vi "LogMessage.vi"(0 "GenericCanAdapterClass in":refnum<class "GenericCanAdapterClass.lvclass">, 1 "LogSuspend":bool, 3 "Name":string, 5 "Arbitration Id":u32 format="%08x", 7 "DataLength":u8, 9 "Data":u8[](array[numeric]) format="%02x", 11 "error in":errorcluster) -> (4 "GenericCanAdapterClass out":refnum<class "GenericCanAdapterClass.lvclass">, 15 "error out":errorcluster)   [LabVIEW 2011, in "GenericCanAdapterClass.lvclass"]
uses:
  GenericCanAdapterClass.lvclass
  GenericCanAdapterClass.lvclass/GenericCanAdapterClass.ctl
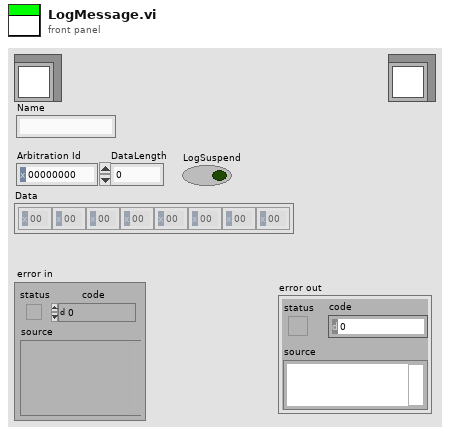
[diagram p1: front panel]
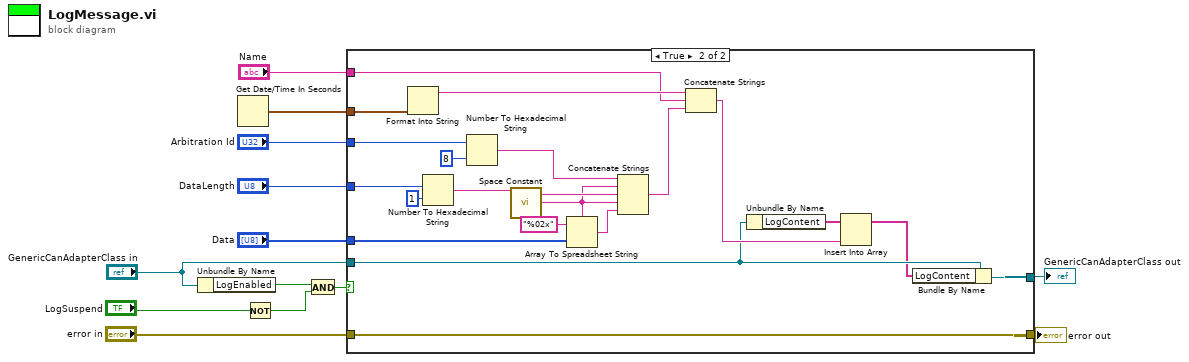
[diagram p0: block diagram]
diagram:
  n1 = Unbundle By Name("GenericCanAdapterClass in") -> ("LogEnabled"=w8:bool)
  n2 = Get Date/Time In Seconds() -> (seconds since 1Jan1904=w13:timestamp)
  n3 = Not(x="LogSuspend") -> (.not. x?=w10:bool)
  n4 = And(x=w8, y=w10) -> (x .and. y?=w11:bool)
  n5 = case shown="True" w11 {
    tunnel: "error in" -> [w15 w22]
    tunnel: [w15 w22] -> w5
    tunnel: [w14 w19] -> w2
    tunnel: "GenericCanAdapterClass in" -> [w14 w18]
    tunnel: "Data" -> [_ w29]
    tunnel: "DataLength" -> [_ w28]
    tunnel: "Arbitration Id" -> [_ w26]
    tunnel: w13 -> [_ w24]
    tunnel: "Name" -> [_ w16]
    frame False {
    }
    frame True {
      n6 = Format Into String(w24) -> (resulting string=w23:string)  [unwired: 3 in, 1 out]
      n7 = Number To Hexadecimal String(1:i16 1 ("width (-)"), 2:w28) -> (0:w35:string)
      n8 = Number To Hexadecimal String(1:i16 8 ("width (-)"), 2:w26) -> (0:w25:string)
      n9 = call <vilib>:"Space Constant.vi"() -> ("String"=w33:string)
      n10 = Array To Spreadsheet String(delimiter (Tab)=w33, array=w29, 3:"%02x" ("format string")) -> (spreadsheet string=w32:string)
      n11 = Concatenate Strings(w25, w33, w35, w33, w32) -> (w30:string)
      n12 = Concatenate Strings(w23, w16, w30) -> (w20:string)
      n13 = Unbundle By Name(w18) -> ("LogContent"=w21:string[])
      n14 = Insert Into Array(array=w21, new element=w20) -> (w17:string[])  [unwired: 1 in]
      n15 = Bundle By Name(cluster=w18, "LogContent"=w17) -> (w19:refnum<class "GenericCanAdapterClass.lvclass">)
    }
  }
  "error out" <- w5
  "GenericCanAdapterClass out" <- w2
